vi "ReadPicoTDMS.vi"() -> ()   [LabVIEW 2010]
panel:
  out "element 0":waveform(dbl)
  out "channel name(s) out":string[](array[string])
  out "group name out":string
  in  "Input file Offset":i64 format="%-#.6p"
  in  "Over Ride Offset":bool
  out "File Offset":i64 format="%-#.6p"
  out "end of file?":bool
  in  "Reset Offset":bool
  in  "count (Samples to read)":i64=20000000 format="%-#.6p"
  out "Waveform Graph":waveform(dbl)[](graph)
  in  "group name in":string
  in  "Data file":path=path "C:/SDK_Repos/picosdk-ni-labview-examples/ps4000a/PicoScope4000aExampleStreaming ChA Data.tdms"
  # "When run the vi reads the number of \"count\" samples\nin the file offset by \"File offset\"\nRepeatly running the example adds the\n\"count\" to the \"File Offset\".\n\n-Use \"Reset OffSet\" button to set \"File Offset\" back to zero.\n\n-Use \"Over ride Offset\" to ironge the File Offset value and read from the start of the file."
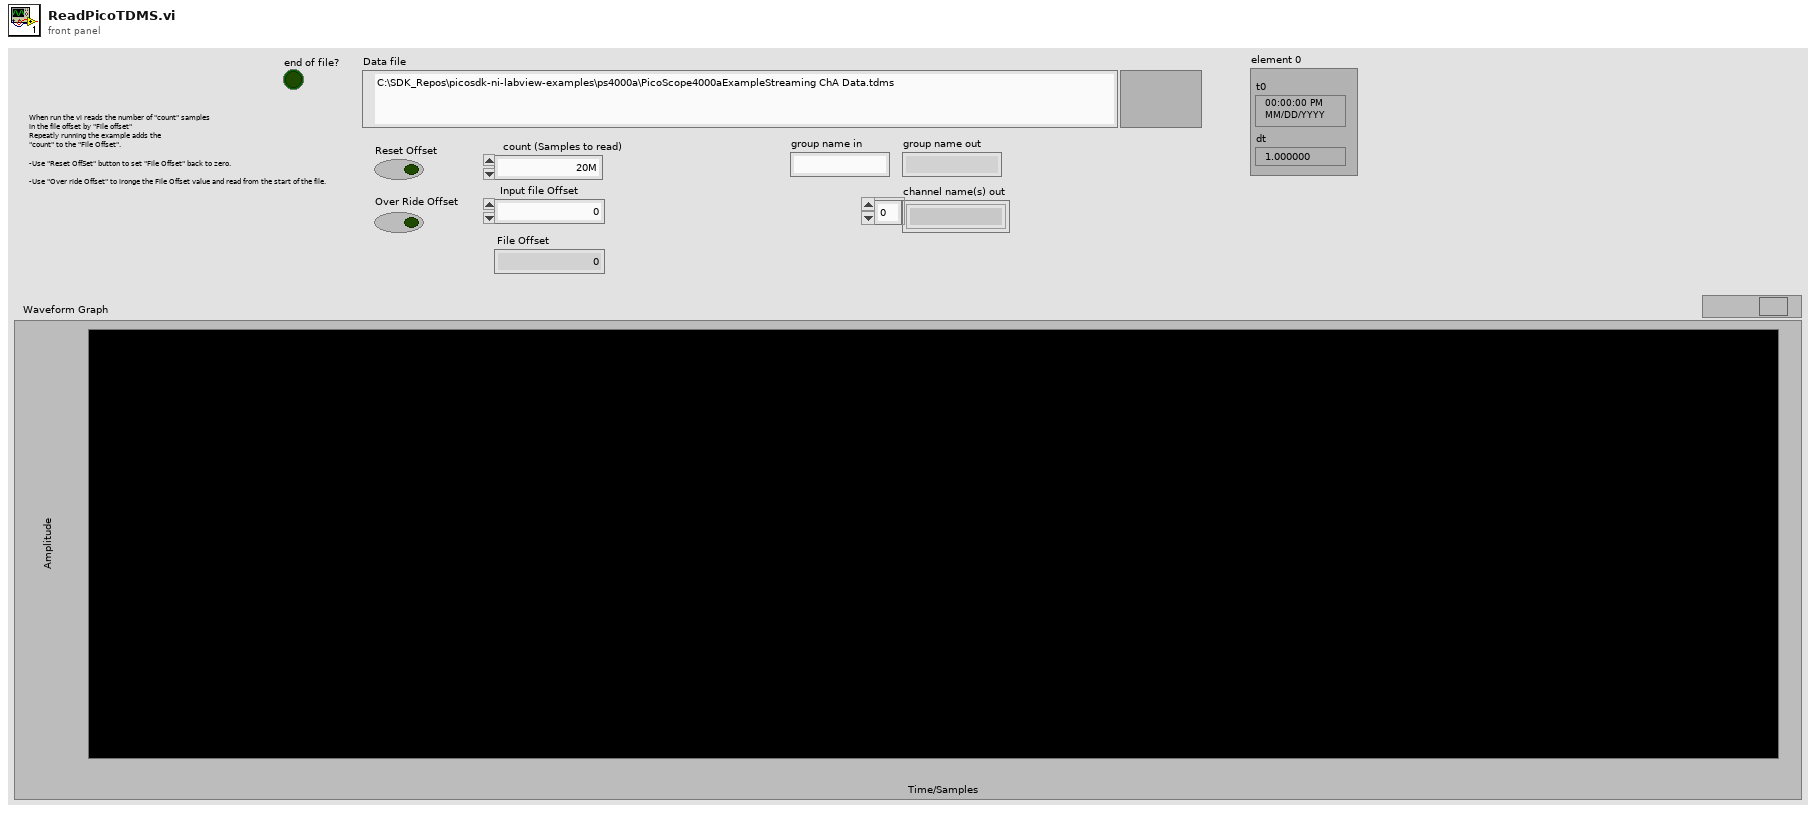
[diagram p1: front panel]
types:
  T1 = enum16{"open", "open or create", "create or replace", "create", "open (read-only)"}
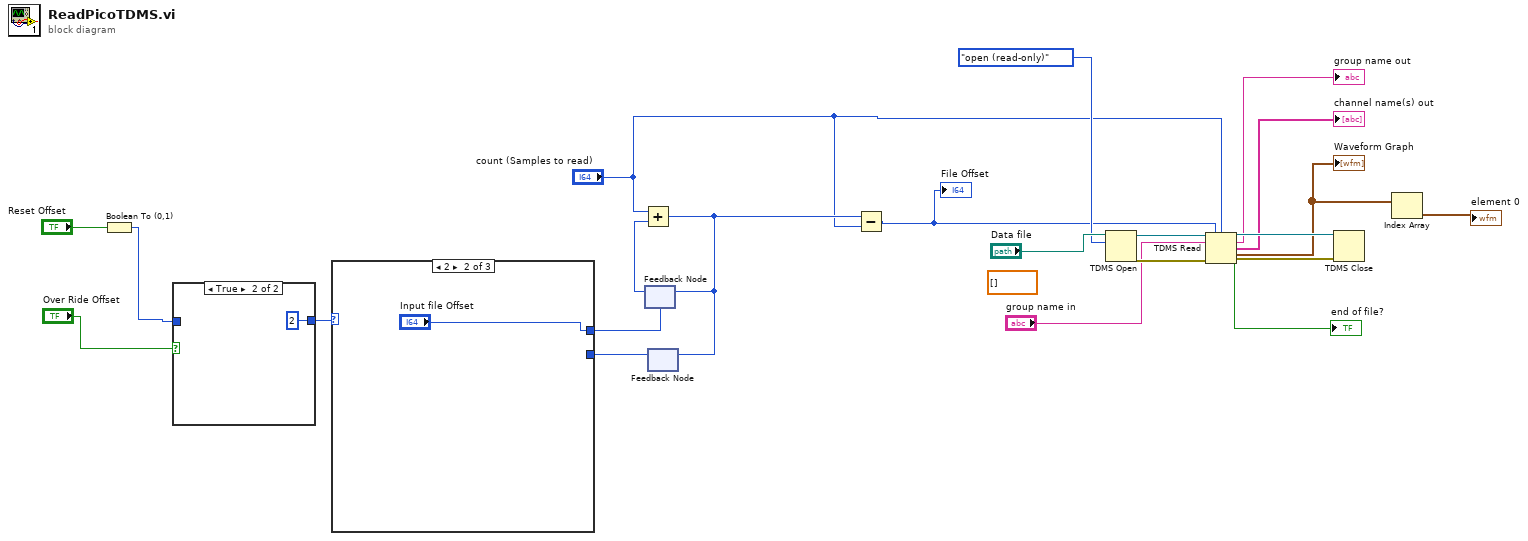
[diagram p0: block diagram]
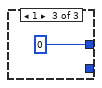
[diagram p4: hidden frame]
diagram:
  (unwired) dbl[] [] ("History Data")
  n1 = Boolean To (0,1)(Boolean="Reset Offset") -> (0, 1=w5:i16)
  n2 = case shown="True" "Over Ride Offset" {
    tunnel: [w23 i16 2] -> w6
    tunnel: w5 -> [w23 _]
    frame False {
    }
    frame True {
    }
  }
  n3 = feedback #1() -> (w14:i64)  [unwired: 1 in]
  n4 = case shown="2" w6 {
    tunnel: [w25 "Input file Offset" i64 0] -> w15
    tunnel: w14 -> [w25 _ _]
    frame 0, Default {
    }
    frame 2 {
    }
    frame 1 {
    }
  }
  n5 = feedback #2(w15) -> (w16:i64)
  n6 = Add(x="count (Samples to read)", y=w16) -> (x+y=w11:i64)
  n7 = feedback-in #2(w11) -> ()
  n8 = feedback-in #1(w11) -> ()
  n9 = Subtract(x=w11, y="count (Samples to read)") -> (x-y=w10:i64)
  "File Offset" <- w10
  n10 = TDMS Open(10:T1."open (read-only)" ("operation (0:open)"), 11:"Data file") -> (0:w21:errorcluster, 3:w17:refnum<k34>)  [unwired: 4 in]
  n11 = TDMS Read(0:w17, 1:w10, 2:"count (Samples to read)", 5:"group name in", 11:w21) -> (4:w18:refnum<k34>, 6:→"group name out":string, 8:→"channel name(s) out":string[], 10:w2:waveform(dbl)[], 14:→"end of file?":bool, 15:w22:errorcluster)  [unwired: 2 in]
  "Waveform Graph" <- w2
  n12 = TDMS Close(8:w22, 11:w18) -> ()  [unwired: 2 out]
  n13 = Index Array(array=w2) -> (element=→"element 0":waveform(dbl))  [unwired: 1 in]
